vi "Init & Start Sequence.vi"(8 "error in (no error)":errorcluster, 9 "Channel Mask":u64, 10 "Config Data":T2, 11 "Connection Data In":T1) -> (0 "error out":errorcluster, 3 "Connection Data Out":T1)   [LabVIEW 2014, in "MSX-E3701_dll.lvlib"]
doc: "Toma los datos de configuracion y su dll se encarga de pasarle los parametros al ADDI-DATA."
uses:
  MSX-E3701_dll.lvlib
  Typedef/Config Data.ctl
  Typedef/Connection Data.ctl
  E:/Repositorio Magnis/INF002/v0/Modules/HAL/Drivers/Sync/ADDI-DATA MSX-E3701/API/MX370x.dll
  MX370x.dll
  E:/Repositorio Magnis/INF002/v0/Modules/HAL/Drivers/Sync/ADDI-DATA MSX-E3701/API/MXCommon.dll
  MXCommon.dll
panel:
  out "Status Sequence":string="Success."
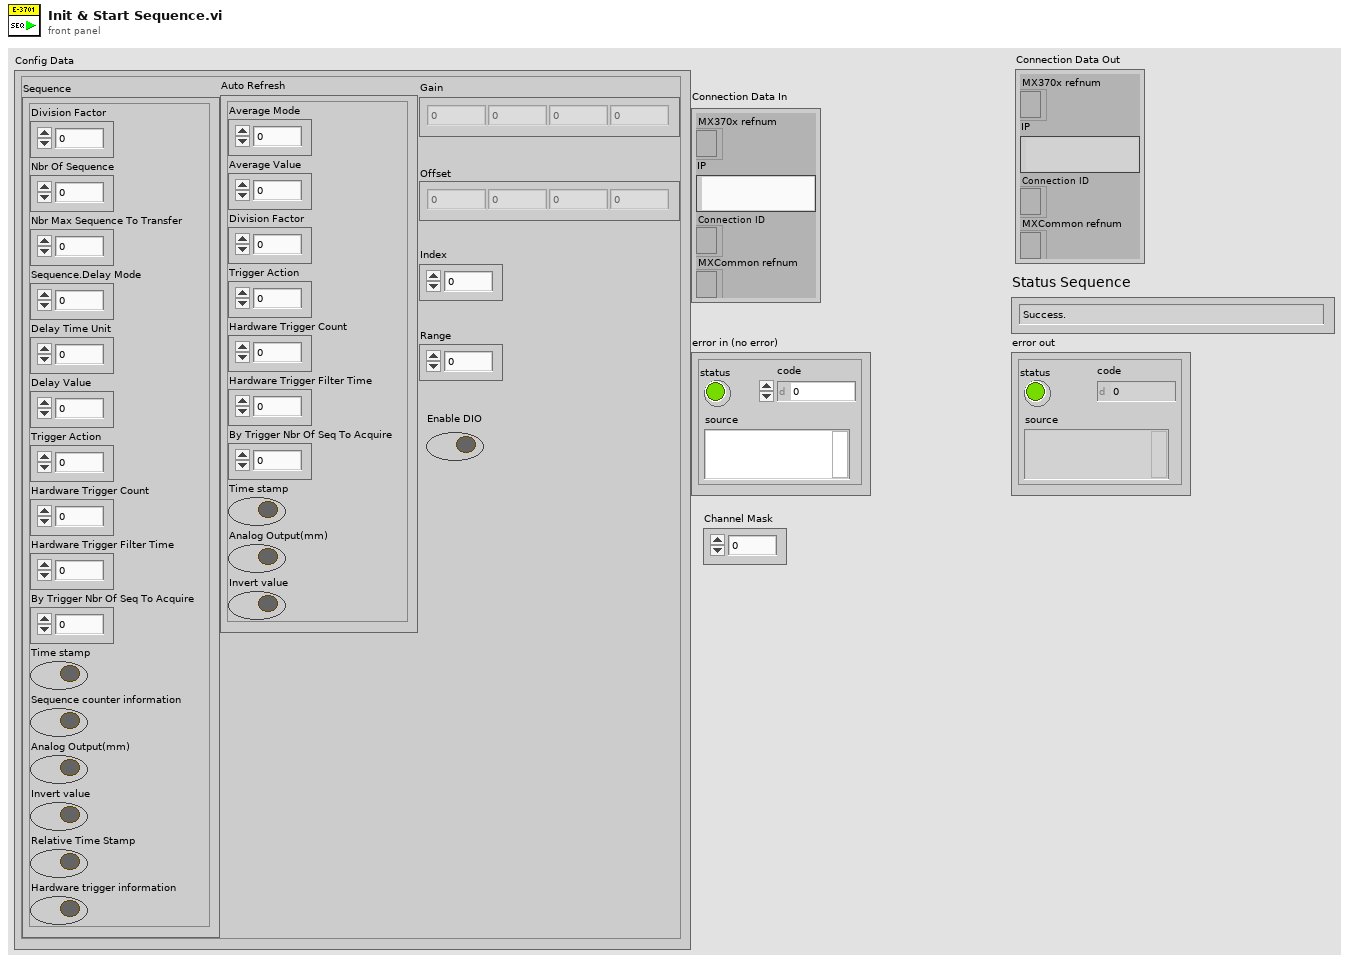
[diagram p1: front panel]
types:
  T1 = typedef "MSX-E3701_dll.lvlib/Connection Data.ctl" = cluster{"MX370x refnum":refnum<k24>, "IP":string, "Connection ID ":refnum<k5>, "MXCommon refnum":refnum<k24>}
  T2 = typedef "MSX-E3701_dll.lvlib/Config Data.ctl" = cluster{"Auto Refresh":cluster{"Average Mode":u64, "Average Value":u64, "Division Factor":u64, "Trigger Action":u64, "Hardware Trigger Count":u64, "Hardware Trigger Filter Time":u64, "By Trigger Nbr Of Seq To Acquire":u64, "Time stamp":bool, "Analog Output(mm)":bool, "Invert value":bool}, "Gain":sgl[], "Offset":sgl[], "Index":u64, "Range":sgl, "Sequence":cluster{"Division Factor":u64, "Nbr Of Sequence":u64, "Nbr Max Sequence To Transfer":u64, "Sequence.Delay Mode":u64, "Delay Time Unit":u64, "Delay Value":u64, "Trigger Action":u64, "Hardware Trigger Count":u64, "Hardware Trigger Filter Time":u64, "By Trigger Nbr Of Seq To Acquire":u64, "Time stamp":bool, "Sequence counter information":bool, "Analog Output(mm)":bool, "Invert value":bool, "Relative Time Stamp":bool, "Hardware trigger information":bool}, "Enable DIO":bool}
  T3 = cluster{"Division Factor":u64, "Nbr Of Sequence":u64, "Nbr Max Sequence To Transfer":u64, "Sequence.Delay Mode":u64, "Delay Time Unit":u64, "Delay Value":u64, "Trigger Action":u64, "Hardware Trigger Count":u64, "Hardware Trigger Filter Time":u64, "By Trigger Nbr Of Seq To Acquire":u64, "Time stamp":bool, "Sequence counter information":bool, "Analog Output(mm)":bool, "Invert value":bool, "Relative Time Stamp":bool, "Hardware trigger information":bool}
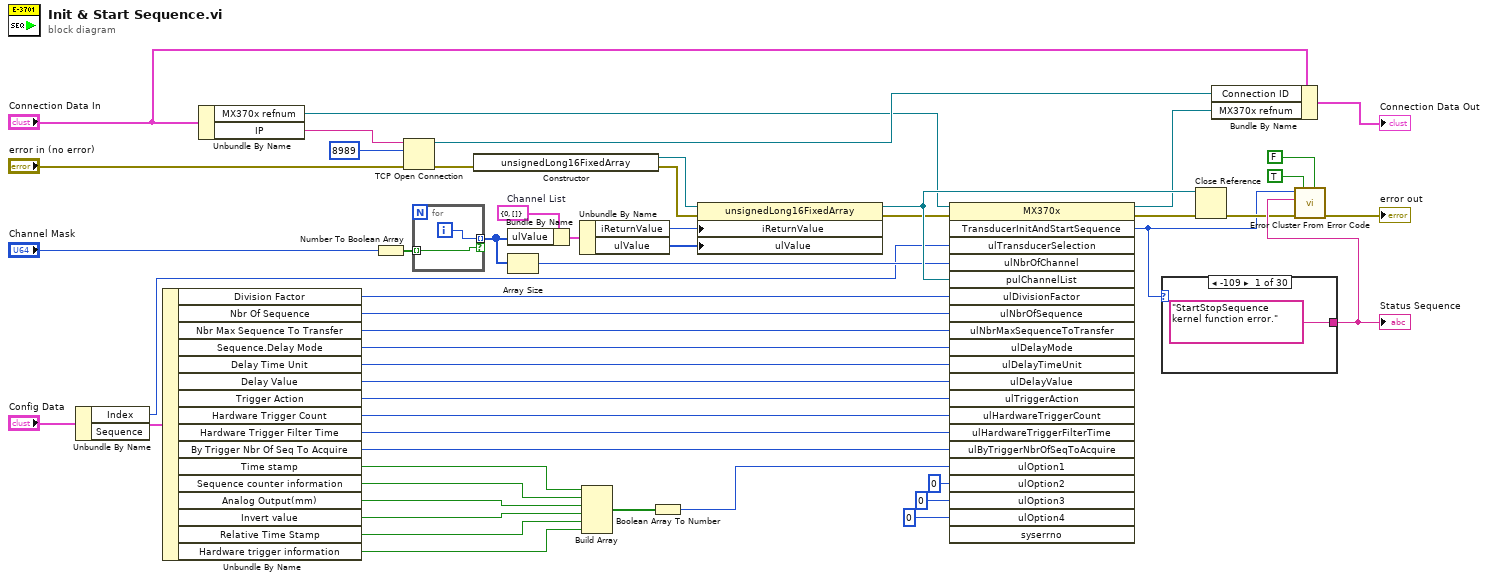
[diagram p0: block diagram]
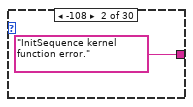
[diagram p2: hidden frame]
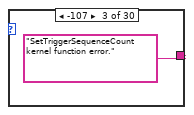
[diagram p3: hidden frame]
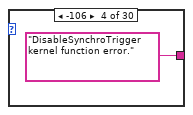
[diagram p4: hidden frame]
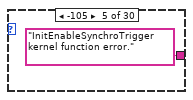
[diagram p5: hidden frame]
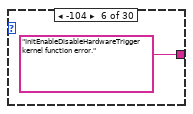
[diagram p6: hidden frame]
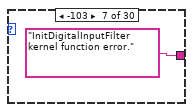
[diagram p7: hidden frame]
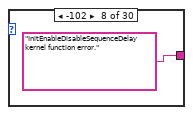
[diagram p8: hidden frame]
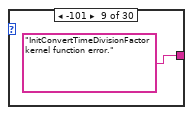
[diagram p9: hidden frame]
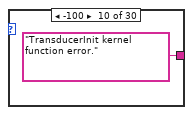
[diagram p10: hidden frame]
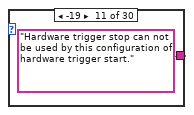
[diagram p11: hidden frame]
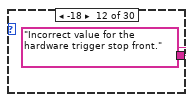
[diagram p12: hidden frame]
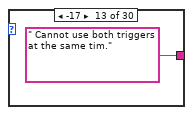
[diagram p13: hidden frame]
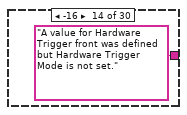
[diagram p14: hidden frame]
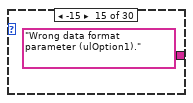
[diagram p15: hidden frame]
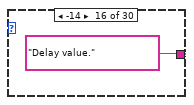
[diagram p16: hidden frame]
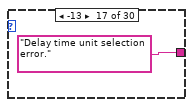
[diagram p17: hidden frame]
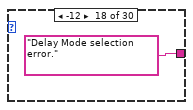
[diagram p18: hidden frame]
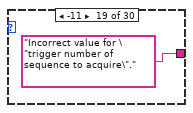
[diagram p19: hidden frame]
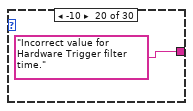
[diagram p20: hidden frame]
diagram:
  w47 = cluster{"iReturnValue":i32, "ulValue":u64[]} {"iReturnValue"=0, "ulValue"=[]}  # Channel List
  n1 = Unbundle By Name("Config Data") -> ("Index"=w1:u64, "Sequence"=w40:T3)
  n2 = Unbundle By Name(w40) -> ("Division Factor"=w39:u64, "Nbr Of Sequence"=w38:u64, "Nbr Max Sequence To Transfer"=w37:u64, "Sequence.Delay Mode"=w36:u64, "Delay Time Unit"=w35:u64, "Delay Value"=w30:u64, "Trigger Action"=w31:u64, "Hardware Trigger Count"=w32:u64, "Hardware Trigger Filter Time"=w33:u64, "By Trigger Nbr Of Seq To Acquire"=w34:u64, "Time stamp"=w24:bool, "Sequence counter information"=w19:bool, "Analog Output(mm)"=w20:bool, "Invert value"=w21:bool, "Relative Time Stamp"=w22:bool, "Hardware trigger information"=w23:bool)
  n3 = Unbundle By Name("Connection Data In") -> ("MX370x refnum"=w4:refnum<k24>, "IP"=w3:string)
  n4 = Number To Boolean Array(number="Channel Mask") -> (Boolean array=w41:bool[])
  n5 = TCP Open Connection(address=w3, remote port or service name=u16 8989 ("Netzwerk-Port"), error in (no error)="error in (no error)") -> (connection ID=w8:refnum<k5>, error out=w7:errorcluster)  [unwired: 2 in]
  n6 = for {
    tunnel: [w54] -> w46 mode=indexing if=w53
    tunnel: w41 -> [w53] mode=indexing
    i -> [w54]
  }
  n7 = constructor class="unsignedLong16FixedArray"(error in=w7) -> (reference out=w52:refnum<k24>, error out=w51:errorcluster)  [unwired: 2 in, 1 out]
  n8 = Bundle By Name(cluster=w47, "ulValue"=w46) -> (w45:cluster{"iReturnValue":i32, "ulValue":u64[]})
  n9 = Array Size(array=w46) -> (size(s)=w44:i32)
  n10 = Unbundle By Name(w45) -> ("iReturnValue"=w43:i32, "ulValue"=w42:u64[])
  n11 = Build Array(w24, w19, w20, w21, w22, w23) -> (w26:bool[])
  n12 = Boolean Array To Number(Boolean array=w26) -> (number=w25:u32)
  n13 = property class="unsignedLong16FixedArray"(reference=w52, error in=w51, "iReturnValue"=w43, "ulValue"=w42) -> (reference out=w50:refnum<k24>, error out=w49:errorcluster)
  n14 = invoke class="MX370x" method="TransducerInitAndStartSequence"(reference=w4, error in=w49, "ulTransducerSelection"=w1, "ulNbrOfChannel"=w44, "pulChannelList"=w50, "ulDivisionFactor"=w39, "ulNbrOfSequence"=w38, "ulNbrMaxSequenceToTransfer"=w37, "ulDelayMode"=w36, "ulDelayTimeUnit"=w35, "ulDelayValue"=w30, "ulTriggerAction"=w31, "ulHardwareTriggerCount"=w32, "ulHardwareTriggerFilterTime"=w33, "ulByTriggerNbrOfSeqToAcquire"=w34, "ulOption1"=w25, "ulOption2"=u64 0, "ulOption3"=u64 0, "ulOption4"=u64 0) -> (reference out=w5:refnum<k24>, error out=w48:errorcluster, "TransducerInitAndStartSequence"=w13:i32)  [unwired: 2 in, 18 out]
  n15 = case shown="-109" w13 {
    tunnel: ["StartStopSequence kernel function error." "InitSequence kernel function error." "SetTriggerSequenceCount kernel function error." "DisableSynchroTrigger kernel function error." "InitEnableSynchroTrigger kernel function error." "InitEnableDisableHardwareTrigger kernel function error." "InitDigitalInputFilter kernel function error." "InitEnableDisableSequenceDelay kernel function error." "InitConvertTimeDivisionFactor kernel function error." "TransducerInit kernel function error." "Hardware trigger stop can not be used by this configuration of hardware trigger start." "Incorrect value for the hardware trigger stop front." " Cannot use both triggers at the same tim." "A value for Hardware Trigger front was defined but Hardware Trigger Mode is not set." "Wrong data format parameter (ulOption1)." "Delay value." "Delay time unit selection error." "Delay Mode selection error." "Incorrect value for \"trigger number of sequence to acquire\"." "Incorrect value for Hardware Trigger filter time." "Incorrect value for Hardware Trigger Count." "Incorrect value for Synchro Trigger Mode." "Incorrect value for Hardware Trigger Front." "Incorrect value for Hardware Trigger Mode." "Division factor error." "Channel array selection error." "Number of channel error." "Transducer selection error." "Means an system error occurred." "Success."] -> w16
    frame -109 {
    }
    frame -108 {
    }
    frame -107 {
    }
    frame -106 {
    }
    frame -105 {
    }
    frame -104 {
    }
    frame -103 {
    }
    frame -102 {
    }
    frame -101 {
    }
    frame -100 {
    }
    frame -19 {
    }
    frame -18 {
    }
    frame -17 {
    }
    frame -16 {
    }
    frame -15 {
    }
    frame -14 {
    }
    frame -13 {
    }
    frame -12 {
    }
    frame -11 {
    }
    frame -10 {
    }
    frame -9 {
    }
    frame -8 {
    }
    frame -7 {
    }
    frame -6 {
    }
    frame -5 {
    }
    frame -4 {
    }
    frame -3 {
    }
    frame -2 {
    }
    frame -1 {
    }
    frame 0, Default {
    }
  }
  "Status Sequence" <- w16
  n16 = Close Reference(reference=w50, error in (no error)=w48) -> (error out=w15:errorcluster)
  n17 = Bundle By Name(cluster="Connection Data In", "Connection ID"=w8, "MX370x refnum"=w5) -> (→"Connection Data Out":T1)
  n18 = call <vilib>:"Error Cluster From Error Code.vi"("is warning? (False)"=FALSE, "show call chain? (False)"=TRUE, "error in (no error)"=w15, "error message (\"\")"=w16, "error code (0)"=w13) -> ("error out"=→"error out":errorcluster)  [unwired: 4 in]
